vi "get_samples.vi"(0 "elemszam":i32, 1 "VISA Refnum in":refnum<visa-resource-name>, 2 "error in (no error)":errorcluster) -> (3 "in samples":u16[](array[numeric]), 4 "out samples":u16[](array[numeric]), 5 "VISA Refnum out":refnum<visa-resource-name>, 6 "error out":errorcluster)   [LabVIEW 2014]
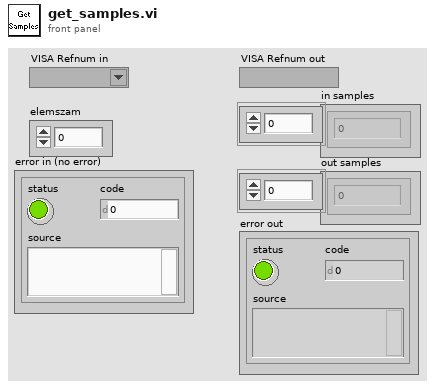
[diagram p1: front panel]
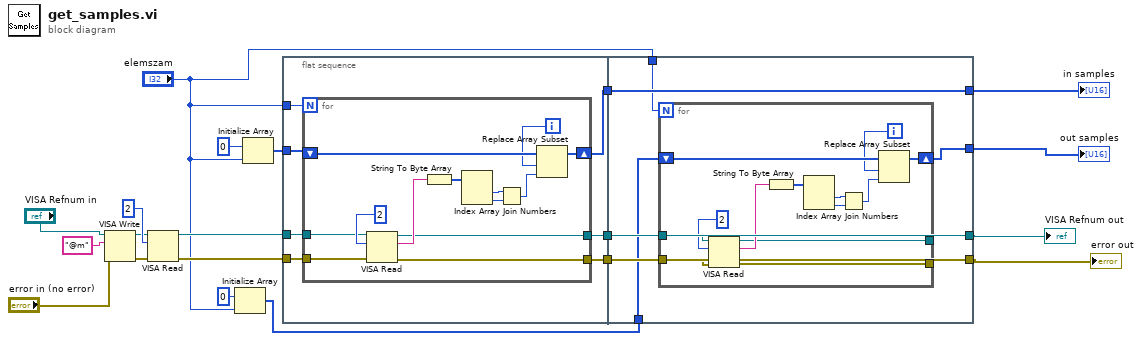
[diagram p0: block diagram]
diagram:
  n1 = VISA Write(VISA resource name="VISA Refnum in", write buffer="@m", error in (no error)="error in (no error)") -> (VISA resource name out=w16:refnum<visa-resource-name>, error out=w17:errorcluster)  [unwired: 1 out]
  n2 = VISA Read(VISA resource name=w16, byte count=u32 2, error in (no error)=w17) -> (VISA resource name out=w12:refnum<visa-resource-name>, error out=w11:errorcluster)  [unwired: 2 out]
  n3 = Initialize Array(0, "elemszam") -> (w3:i32[])
  n4 = Initialize Array(0, "elemszam") -> (w10:i32[])
  n5 = flat-sequence {
    tunnel: w12 -> [w26]
    tunnel: w11 -> [w25]
    tunnel: w10 -> [w24]
    tunnel: "elemszam" -> [w21]
    tunnel: [w27] -> w9
    tunnel: [w23] -> w8
    tunnel: [w22] -> w7
    tunnel: [w43] -> w4
    tunnel: [w44] -> w5
    tunnel: [w46] -> w14
    tunnel: w9 -> [w46]
    tunnel: w8 -> [w44]
    tunnel: w7 -> [w43]
    tunnel: [w45] -> w6
    tunnel: w3 -> [w42]
    tunnel: "elemszam" -> [w41]
    frame #0 {
      n6 = for {
        N: w21 -> [_]
        shift-right: [w34] -> w27
        shift-left: w24 -> [w35]
        tunnel: w26 -> [w32]
        tunnel: w25 -> [w31]
        tunnel: [w29] -> w23
        tunnel: [w28] -> w22
        i -> [w30]
        n7 = VISA Read(VISA resource name=w32, byte count=u32 2, error in (no error)=w31) -> (VISA resource name out=w29:refnum<visa-resource-name>, read buffer=w37:string, error out=w28:errorcluster)  [unwired: 1 out]
        n8 = String To Byte Array(string=w37) -> (unsigned byte array=w36:u8[])
        n9 = Index Array(array=w36) -> (element #1=w39:u8, element #2=w38:u8)  [unwired: 2 in]
        n10 = Join Numbers(hi=w39, lo=w38) -> ((hi.lo)=w33:u16)
        n11 = Replace Array Subset(array=w35, new element=w33, index=w30) -> (w34:i32[])
      }
    }
    frame #1 {
      n12 = for {
        N: w41 -> [_]
        shift-right: [w53] -> w45
        shift-left: w42 -> [w54]
        tunnel: [w50] -> _
        tunnel: [w49] -> _
        tunnel: w44 -> [w48]
        tunnel: w43 -> [w47]
        i -> [w51]
        n13 = VISA Read(VISA resource name=w48, byte count=u32 2, error in (no error)=w47) -> (VISA resource name out=w50:refnum<visa-resource-name>, read buffer=w56:string, error out=w49:errorcluster)  [unwired: 1 out]
        n14 = String To Byte Array(string=w56) -> (unsigned byte array=w55:u8[])
        n15 = Index Array(array=w55) -> (element #1=w58:u8, element #2=w57:u8)  [unwired: 2 in]
        n16 = Join Numbers(hi=w58, lo=w57) -> ((hi.lo)=w52:u16)
        n17 = Replace Array Subset(array=w54, new element=w52, index=w51) -> (w53:i32[])
      }
    }
  }
  "error out" <- w4
  "VISA Refnum out" <- w5
  "in samples" <- w14
  "out samples" <- w6
